vi "Read datatype.vi"(8 "error in (no error)":errorcluster, 11 "JSON Boolean in":refnum<class "JSON Boolean.lvclass">) -> (0 "error out":errorcluster, 2 "datatype":T1, 3 "JSON Boolean out":refnum<class "JSON Boolean.lvclass">)   [LabVIEW 2017, in "LVJSON.lvlib" / "JSON Boolean.lvclass"]
uses:
  JSON Boolean.lvclass
  JSON Types.ctl
  LVJSON.lvlib
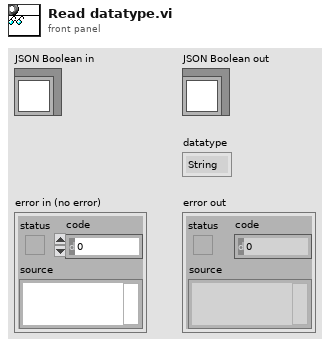
[diagram p1: front panel]
types:
  T1 = typedef "LVJSON.lvlib/JSON Types.ctl" = enum16{"String", "Numeric", "Boolean", "NULL", "Object", "1D Array", "Unknown"}
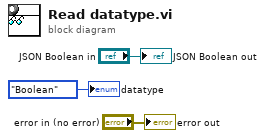
[diagram p0: block diagram]
diagram:
  "error out" <- "error in (no error)"
  "JSON Boolean out" <- "JSON Boolean in"
  "datatype" <- JSON_Types."Boolean" ("datatype")
